vi "Pose3d_RotationVectorToMatrix.vi"(11 "RotationVector":dbl[](array[numeric])) -> (3 "Rotation Matrix":T1)   [LabVIEW 2019, in "Trajectory_Library.lvlib"]
doc: "Applies the hat operator to a rotation vector.\n \nIt takes a rotation vector and returns the corresponding matrix representation of the Lie algebra element (a 3x3 rotation matrix).\n \n\nParameters:\n - RotationVector -- rotation The rotation vector.\n\nReturn:\n - RotationMatrix -- The rotation vector as a 3x3 rotation matrix."
uses:
  Trajectory_Library.lvlib
  <vilib>/Analysis/Matrix/Datatypes/RealMatrix.ctl
  <vilib>/Analysis/Matrix/NI_Matrix.lvlib
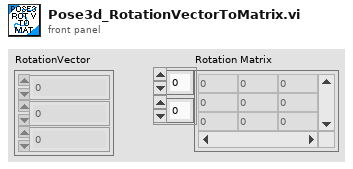
[diagram p1: front panel]
types:
  T1 = typedef "NI_Matrix.lvlib/RealMatrix.ctl" = dbl[][]
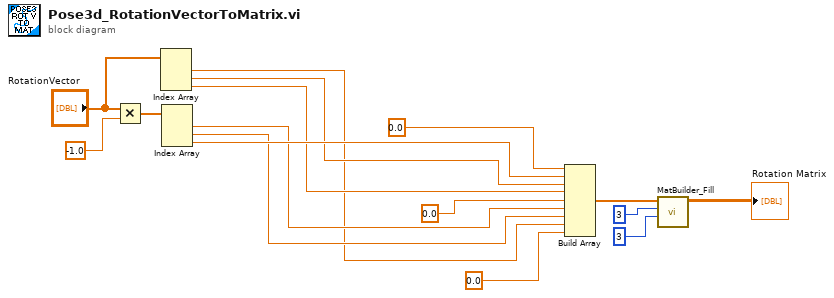
[diagram p0: block diagram]
diagram:
  n1 = Multiply(x="RotationVector", y=-1.0) -> (x*y=w8:dbl[])
  n2 = Index Array(array="RotationVector") -> (element #1=w1:dbl, element #2=w5:dbl, element #3=w4:dbl)  [unwired: 3 in]
  n3 = Index Array(array=w8) -> (element #1=w3:dbl, element #2=w2:dbl, element #3=w6:dbl)  [unwired: 3 in]
  n4 = Build Array(0.0 ("element"), w6, w5, w4, 0.0 ("element"), w3, w2, w1, 0.0 ("element")) -> (w13:dbl[])
  n5 = call "MatBuilder_Fill.vi"("Columns"=3, "Rows"=3, "Value List"=w13) -> ("output matrix"=→"Rotation Matrix":T1)  [unwired: 8 in]
